vi "PART1.vi"() -> ()   [LabVIEW 2019]
uses:
  <vilib>/rvi/eio/common/nirviEmuTemplateMethod_errors.vi
  <vilib>/eio/EIONode/EIONode.xnode
  <vilib>/eio/EIOMethodNode/EIOMethodNode.xnode
panel:
  out "SDA 11":bool
  out "SDA 10":bool
  out "SDA 9":bool
  out "SDA 8":bool
  out "SDA 7":bool
  out "SDA 6":bool
  out "SDA 5":bool
  out "SDA 4":bool
  out "SDA 3":bool
  out "SDA 2":bool
  out "SDA":bool
diagram:
  n1 = flat-sequence {
    frame #0 {
      n2 = xnode "FPGA I/O Node"("SDA"=FALSE) -> ()  [unwired: 1 in, 1 out]
      n3 = xnode "FPGA I/O Node"("SCL"=TRUE) -> ()  [unwired: 1 in, 1 out]
    }
    frame #1 {
      n4 = call "Wait3"("Count(mSec)"=u32 100) -> ()  [unwired: 1 out]
    }
    frame #2 {
      n5 = xnode "FPGA I/O Node"("SCL"=FALSE) -> ()  [unwired: 1 in, 1 out]
    }
    frame #3 {
      n6 = call "Wait"("Count(mSec)"=u32 100) -> ()  [unwired: 1 out]
    }
    frame #4 {
      # "bit 0"
      n7 = xnode "FPGA I/O Node"("SDA"=FALSE) -> ()  [unwired: 1 in, 1 out]
    }
    frame #5 {
      n8 = xnode "FPGA I/O Node"("SCL"=TRUE) -> ()  [unwired: 1 in, 1 out]
    }
    frame #6 {
      n9 = call "Wait2"("Count(mSec)"=u32 100) -> ()  [unwired: 1 out]
    }
    frame #7 {
      n10 = xnode "FPGA I/O Node"("SCL"=FALSE) -> ()  [unwired: 1 in, 1 out]
    }
    frame #8 {
      n11 = call "Wait4"("Count(mSec)"=u32 100) -> ()  [unwired: 1 out]
    }
    frame #9 {
      # "bit 0"
      n12 = xnode "FPGA I/O Node"("SDA"=FALSE) -> ()  [unwired: 1 in, 1 out]
    }
    frame #10 {
      n13 = xnode "FPGA I/O Node"("SCL"=TRUE) -> ()  [unwired: 1 in, 1 out]
    }
    frame #11 {
      n14 = call "Wait6"("Count(mSec)"=u32 100) -> ()  [unwired: 1 out]
    }
    frame #12 {
      n15 = xnode "FPGA I/O Node"("SCL"=FALSE) -> ()  [unwired: 1 in, 1 out]
    }
    frame #13 {
      n16 = call "Wait5"("Count(mSec)"=u32 100) -> ()  [unwired: 1 out]
    }
    frame #14 {
      # "bit 1"
      n17 = xnode "FPGA I/O Node"("SDA"=TRUE) -> ()  [unwired: 1 in, 1 out]
    }
    frame #15 {
      n18 = xnode "FPGA I/O Node"("SCL"=TRUE) -> ()  [unwired: 1 in, 1 out]
    }
    frame #16 {
      n19 = call "Wait7"("Count(mSec)"=u32 100) -> ()  [unwired: 1 out]
    }
    frame #17 {
      n20 = xnode "FPGA I/O Node"("SCL"=FALSE) -> ()  [unwired: 1 in, 1 out]
    }
    frame #18 {
      n21 = call "Wait8"("Count(mSec)"=u32 100) -> ()  [unwired: 1 out]
    }
    frame #19 {
      # "bit 1"
      n22 = xnode "FPGA I/O Node"("SDA"=TRUE) -> ()  [unwired: 1 in, 1 out]
    }
    frame #20 {
      n23 = xnode "FPGA I/O Node"("SCL"=TRUE) -> ()  [unwired: 1 in, 1 out]
    }
    frame #21 {
      n24 = call "Wait9"("Count(mSec)"=u32 100) -> ()  [unwired: 1 out]
    }
    frame #22 {
      n25 = xnode "FPGA I/O Node"("SCL"=FALSE) -> ()  [unwired: 1 in, 1 out]
    }
    frame #23 {
      n26 = call "Wait10"("Count(mSec)"=u32 100) -> ()  [unwired: 1 out]
    }
    frame #24 {
      # "bit 0"
      n27 = xnode "FPGA I/O Node"("SDA"=FALSE) -> ()  [unwired: 1 in, 1 out]
    }
    frame #25 {
      n28 = xnode "FPGA I/O Node"("SCL"=TRUE) -> ()  [unwired: 1 in, 1 out]
    }
    frame #26 {
      n29 = call "Wait11"("Count(mSec)"=u32 100) -> ()  [unwired: 1 out]
    }
    frame #27 {
      n30 = xnode "FPGA I/O Node"("SCL"=FALSE) -> ()  [unwired: 1 in, 1 out]
    }
    frame #28 {
      n31 = call "Wait12"("Count(mSec)"=u32 100) -> ()  [unwired: 1 out]
    }
    frame #29 {
      # "bit 0"
      n32 = xnode "FPGA I/O Node"("SDA"=FALSE) -> ()  [unwired: 1 in, 1 out]
    }
    frame #30 {
      n33 = xnode "FPGA I/O Node"("SCL"=TRUE) -> ()  [unwired: 1 in, 1 out]
    }
    frame #31 {
      n34 = call "Wait13"("Count(mSec)"=u32 100) -> ()  [unwired: 1 out]
    }
    frame #32 {
      n35 = xnode "FPGA I/O Node"("SCL"=FALSE) -> ()  [unwired: 1 in, 1 out]
    }
    frame #33 {
      n36 = call "Wait14"("Count(mSec)"=u32 100) -> ()  [unwired: 1 out]
    }
    frame #34 {
      # "bit 1"
      n37 = xnode "FPGA I/O Node"("SDA"=TRUE) -> ()  [unwired: 1 in, 1 out]
    }
    frame #35 {
      n38 = xnode "FPGA I/O Node"("SCL"=TRUE) -> ()  [unwired: 1 in, 1 out]
    }
    frame #36 {
      n39 = call "Wait15"("Count(mSec)"=u32 100) -> ()  [unwired: 1 out]
    }
    frame #37 {
      n40 = xnode "FPGA I/O Node"("SCL"=FALSE) -> ()  [unwired: 1 in, 1 out]
    }
    frame #38 {
      n41 = call "Wait16"("Count(mSec)"=u32 100) -> ()  [unwired: 1 out]
    }
    frame #39 {
      # "bit 0"
      n42 = xnode "FPGA I/O Node"("SDA"=FALSE) -> ()  [unwired: 1 in, 1 out]
    }
    frame #40 {
      n43 = xnode "FPGA I/O Node"("SCL"=TRUE) -> ()  [unwired: 1 in, 1 out]
    }
    frame #41 {
      n44 = call "Wait17"("Count(mSec)"=u32 100) -> ()  [unwired: 1 out]
    }
    frame #42 {
      n45 = xnode "FPGA I/O Node"("SCL"=FALSE) -> ()  [unwired: 1 in, 1 out]
    }
    frame #43 {
      n46 = call "Wait18"("Count(mSec)"=u32 100) -> ()  [unwired: 1 out]
    }
    frame #44 {
      n47 = flat-sequence {
        frame #0 {
          n48 = xnode "FPGA I/O Method Node"("Enable"=FALSE) -> ()  [unwired: 1 in, 1 out]
        }
        frame #1 {
          # "Read ACK"
          n49 = xnode "FPGA I/O Node"() -> ("SDA"=→"SDA":bool)  [unwired: 1 in, 1 out]
        }
      }
    }
    frame #45 {
      n50 = xnode "FPGA I/O Node"("SCL"=TRUE) -> ()  [unwired: 1 in, 1 out]
    }
    frame #46 {
      n51 = call "Wait19"("Count(mSec)"=u32 100) -> ()  [unwired: 1 out]
    }
    frame #47 {
      n52 = xnode "FPGA I/O Node"("SCL"=FALSE) -> ()  [unwired: 1 in, 1 out]
    }
    frame #48 {
      n53 = call "Wait20"("Count(mSec)"=u32 100) -> ()  [unwired: 1 out]
    }
    frame #49 {
      # "bit 0"
      n54 = xnode "FPGA I/O Node"("SDA"=FALSE) -> ()  [unwired: 1 in, 1 out]
    }
    frame #50 {
      n55 = xnode "FPGA I/O Node"("SCL"=TRUE) -> ()  [unwired: 1 in, 1 out]
    }
    frame #51 {
      n56 = call "Wait21"("Count(mSec)"=u32 100) -> ()  [unwired: 1 out]
    }
    frame #52 {
      n57 = xnode "FPGA I/O Node"("SCL"=FALSE) -> ()  [unwired: 1 in, 1 out]
    }
    frame #53 {
      n58 = call "Wait22"("Count(mSec)"=u32 100) -> ()  [unwired: 1 out]
    }
    frame #54 {
      # "bit 1"
      n59 = xnode "FPGA I/O Node"("SDA"=TRUE) -> ()  [unwired: 1 in, 1 out]
    }
    frame #55 {
      n60 = xnode "FPGA I/O Node"("SCL"=TRUE) -> ()  [unwired: 1 in, 1 out]
    }
    frame #56 {
      n61 = call "Wait23"("Count(mSec)"=u32 100) -> ()  [unwired: 1 out]
    }
    frame #57 {
      n62 = xnode "FPGA I/O Node"("SCL"=FALSE) -> ()  [unwired: 1 in, 1 out]
    }
    frame #58 {
      n63 = call "Wait24"("Count(mSec)"=u32 100) -> ()  [unwired: 1 out]
    }
    frame #59 {
      # "bit 0"
      n64 = xnode "FPGA I/O Node"("SDA"=FALSE) -> ()  [unwired: 1 in, 1 out]
    }
    frame #60 {
      n65 = xnode "FPGA I/O Node"("SCL"=TRUE) -> ()  [unwired: 1 in, 1 out]
    }
    frame #61 {
      n66 = call "Wait25"("Count(mSec)"=u32 100) -> ()  [unwired: 1 out]
    }
    frame #62 {
      n67 = xnode "FPGA I/O Node"("SCL"=FALSE) -> ()  [unwired: 1 in, 1 out]
    }
    frame #63 {
      n68 = call "Wait26"("Count(mSec)"=u32 100) -> ()  [unwired: 1 out]
    }
    frame #64 {
      # "bit 1"
      n69 = xnode "FPGA I/O Node"("SDA"=TRUE) -> ()  [unwired: 1 in, 1 out]
    }
    frame #65 {
      n70 = xnode "FPGA I/O Node"("SCL"=TRUE) -> ()  [unwired: 1 in, 1 out]
    }
    frame #66 {
      n71 = call "Wait27"("Count(mSec)"=u32 100) -> ()  [unwired: 1 out]
    }
    frame #67 {
      n72 = xnode "FPGA I/O Node"("SCL"=FALSE) -> ()  [unwired: 1 in, 1 out]
    }
    frame #68 {
      n73 = call "Wait28"("Count(mSec)"=u32 100) -> ()  [unwired: 1 out]
    }
    frame #69 {
      # "bit 0"
      n74 = xnode "FPGA I/O Node"("SDA"=FALSE) -> ()  [unwired: 1 in, 1 out]
    }
    frame #70 {
      n75 = xnode "FPGA I/O Node"("SCL"=TRUE) -> ()  [unwired: 1 in, 1 out]
    }
    frame #71 {
      n76 = call "Wait29"("Count(mSec)"=u32 100) -> ()  [unwired: 1 out]
    }
    frame #72 {
      n77 = xnode "FPGA I/O Node"("SCL"=FALSE) -> ()  [unwired: 1 in, 1 out]
    }
    frame #73 {
      n78 = call "Wait30"("Count(mSec)"=u32 100) -> ()  [unwired: 1 out]
    }
    frame #74 {
      # "bit 0"
      n79 = xnode "FPGA I/O Node"("SDA"=FALSE) -> ()  [unwired: 1 in, 1 out]
    }
    frame #75 {
      n80 = xnode "FPGA I/O Node"("SCL"=TRUE) -> ()  [unwired: 1 in, 1 out]
    }
    frame #76 {
      n81 = call "Wait31"("Count(mSec)"=u32 100) -> ()  [unwired: 1 out]
    }
    frame #77 {
      n82 = xnode "FPGA I/O Node"("SCL"=FALSE) -> ()  [unwired: 1 in, 1 out]
    }
    frame #78 {
      n83 = call "Wait32"("Count(mSec)"=u32 100) -> ()  [unwired: 1 out]
    }
    frame #79 {
      # "bit 1"
      n84 = xnode "FPGA I/O Node"("SDA"=TRUE) -> ()  [unwired: 1 in, 1 out]
    }
    frame #80 {
      n85 = xnode "FPGA I/O Node"("SCL"=TRUE) -> ()  [unwired: 1 in, 1 out]
    }
    frame #81 {
      n86 = call "Wait33"("Count(mSec)"=u32 100) -> ()  [unwired: 1 out]
    }
    frame #82 {
      n87 = xnode "FPGA I/O Node"("SCL"=FALSE) -> ()  [unwired: 1 in, 1 out]
    }
    frame #83 {
      n88 = call "Wait34"("Count(mSec)"=u32 100) -> ()  [unwired: 1 out]
    }
    frame #84 {
      n89 = flat-sequence {
        frame #0 {
          n90 = xnode "FPGA I/O Method Node"("Enable"=FALSE) -> ()  [unwired: 1 in, 1 out]
        }
        frame #1 {
          # "Read ACK"
          n91 = xnode "FPGA I/O Node"() -> ("SDA"=→"SDA 2":bool)  [unwired: 1 in, 1 out]
        }
      }
    }
    frame #85 {
      n92 = xnode "FPGA I/O Node"("SDA"=FALSE) -> ()  [unwired: 1 in, 1 out]
      n93 = xnode "FPGA I/O Node"("SCL"=TRUE) -> ()  [unwired: 1 in, 1 out]
    }
    frame #86 {
      n94 = call "Wait35"("Count(mSec)"=u32 100) -> ()  [unwired: 1 out]
    }
    frame #87 {
      n95 = xnode "FPGA I/O Node"("SCL"=FALSE) -> ()  [unwired: 1 in, 1 out]
    }
    frame #88 {
      n96 = call "Wait36"("Count(mSec)"=u32 100) -> ()  [unwired: 1 out]
    }
    frame #89 {
      # "bit 0"
      n97 = xnode "FPGA I/O Node"("SDA"=FALSE) -> ()  [unwired: 1 in, 1 out]
    }
    frame #90 {
      n98 = xnode "FPGA I/O Node"("SCL"=TRUE) -> ()  [unwired: 1 in, 1 out]
    }
    frame #91 {
      n99 = call "Wait37"("Count(mSec)"=u32 100) -> ()  [unwired: 1 out]
    }
    frame #92 {
      n100 = xnode "FPGA I/O Node"("SCL"=FALSE) -> ()  [unwired: 1 in, 1 out]
    }
    frame #93 {
      n101 = call "Wait38"("Count(mSec)"=u32 100) -> ()  [unwired: 1 out]
    }
    frame #94 {
      # "bit 0"
      n102 = xnode "FPGA I/O Node"("SDA"=FALSE) -> ()  [unwired: 1 in, 1 out]
    }
    frame #95 {
      n103 = xnode "FPGA I/O Node"("SCL"=TRUE) -> ()  [unwired: 1 in, 1 out]
    }
    frame #96 {
      n104 = call "Wait39"("Count(mSec)"=u32 100) -> ()  [unwired: 1 out]
    }
    frame #97 {
      n105 = xnode "FPGA I/O Node"("SCL"=FALSE) -> ()  [unwired: 1 in, 1 out]
    }
    frame #98 {
      n106 = call "Wait40"("Count(mSec)"=u32 100) -> ()  [unwired: 1 out]
    }
    frame #99 {
      # "bit 1"
      n107 = xnode "FPGA I/O Node"("SDA"=TRUE) -> ()  [unwired: 1 in, 1 out]
    }
    frame #100 {
      n108 = xnode "FPGA I/O Node"("SCL"=TRUE) -> ()  [unwired: 1 in, 1 out]
    }
    frame #101 {
      n109 = call "Wait41"("Count(mSec)"=u32 100) -> ()  [unwired: 1 out]
    }
    frame #102 {
      n110 = xnode "FPGA I/O Node"("SCL"=FALSE) -> ()  [unwired: 1 in, 1 out]
    }
    frame #103 {
      n111 = call "Wait42"("Count(mSec)"=u32 100) -> ()  [unwired: 1 out]
    }
    frame #104 {
      # "bit 1"
      n112 = xnode "FPGA I/O Node"("SDA"=TRUE) -> ()  [unwired: 1 in, 1 out]
    }
    frame #105 {
      n113 = xnode "FPGA I/O Node"("SCL"=TRUE) -> ()  [unwired: 1 in, 1 out]
    }
    frame #106 {
      n114 = call "Wait43"("Count(mSec)"=u32 100) -> ()  [unwired: 1 out]
    }
    frame #107 {
      n115 = xnode "FPGA I/O Node"("SCL"=FALSE) -> ()  [unwired: 1 in, 1 out]
    }
    frame #108 {
      n116 = call "Wait44"("Count(mSec)"=u32 100) -> ()  [unwired: 1 out]
    }
    frame #109 {
      # "bit 0"
      n117 = xnode "FPGA I/O Node"("SDA"=FALSE) -> ()  [unwired: 1 in, 1 out]
    }
    frame #110 {
      n118 = xnode "FPGA I/O Node"("SCL"=TRUE) -> ()  [unwired: 1 in, 1 out]
    }
    frame #111 {
      n119 = call "Wait45"("Count(mSec)"=u32 100) -> ()  [unwired: 1 out]
    }
    frame #112 {
      n120 = xnode "FPGA I/O Node"("SCL"=FALSE) -> ()  [unwired: 1 in, 1 out]
    }
    frame #113 {
      n121 = call "Wait46"("Count(mSec)"=u32 100) -> ()  [unwired: 1 out]
    }
    frame #114 {
      # "bit 0"
      n122 = xnode "FPGA I/O Node"("SDA"=FALSE) -> ()  [unwired: 1 in, 1 out]
    }
    frame #115 {
      n123 = xnode "FPGA I/O Node"("SCL"=TRUE) -> ()  [unwired: 1 in, 1 out]
    }
    frame #116 {
      n124 = call "Wait47"("Count(mSec)"=u32 100) -> ()  [unwired: 1 out]
    }
    frame #117 {
      n125 = xnode "FPGA I/O Node"("SCL"=FALSE) -> ()  [unwired: 1 in, 1 out]
    }
    frame #118 {
      n126 = call "Wait48"("Count(mSec)"=u32 100) -> ()  [unwired: 1 out]
    }
    frame #119 {
      # "bit 1"
      n127 = xnode "FPGA I/O Node"("SDA"=TRUE) -> ()  [unwired: 1 in, 1 out]
    }
    frame #120 {
      n128 = xnode "FPGA I/O Node"("SCL"=TRUE) -> ()  [unwired: 1 in, 1 out]
    }
    frame #121 {
      n129 = call "Wait49"("Count(mSec)"=u32 100) -> ()  [unwired: 1 out]
    }
    frame #122 {
      n130 = xnode "FPGA I/O Node"("SCL"=FALSE) -> ()  [unwired: 1 in, 1 out]
    }
    frame #123 {
      n131 = call "Wait50"("Count(mSec)"=u32 100) -> ()  [unwired: 1 out]
    }
    frame #124 {
      # "bit 1"
      n132 = xnode "FPGA I/O Node"("SDA"=TRUE) -> ()  [unwired: 1 in, 1 out]
    }
    frame #125 {
      n133 = xnode "FPGA I/O Node"("SCL"=TRUE) -> ()  [unwired: 1 in, 1 out]
    }
    frame #126 {
      n134 = call "Wait51"("Count(mSec)"=u32 100) -> ()  [unwired: 1 out]
    }
    frame #127 {
      n135 = xnode "FPGA I/O Node"("SCL"=FALSE) -> ()  [unwired: 1 in, 1 out]
    }
    frame #128 {
      # "read ACK"
      n136 = flat-sequence {
        frame #0 {
          n137 = xnode "FPGA I/O Method Node"("Enable"=FALSE) -> ()  [unwired: 1 in, 1 out]
        }
        frame #1 {
          # "Read ACK"
          n138 = xnode "FPGA I/O Node"() -> ("SDA"=→"SDA 3":bool)  [unwired: 1 in, 1 out]
        }
      }
    }
    frame #129 {
      n139 = xnode "FPGA I/O Node"("SCL"=TRUE) -> ()  [unwired: 1 in, 1 out]
    }
    frame #130 {
      n140 = call "Wait52"("Count(mSec)"=u32 100) -> ()  [unwired: 1 out]
    }
    frame #131 {
      n141 = xnode "FPGA I/O Node"("SCL"=FALSE) -> ()  [unwired: 1 in, 1 out]
    }
    frame #132 {
      # "read MSB Data"
      n142 = xnode "FPGA I/O Node"() -> ("SDA"=→"SDA 4":bool)  [unwired: 1 in, 1 out]
    }
    frame #133 {
      n143 = xnode "FPGA I/O Node"("SCL"=TRUE) -> ()  [unwired: 1 in, 1 out]
    }
    frame #134 {
      n144 = call "Wait53"("Count(mSec)"=u32 100) -> ()  [unwired: 1 out]
    }
    frame #135 {
      n145 = xnode "FPGA I/O Node"("SCL"=FALSE) -> ()  [unwired: 1 in, 1 out]
    }
    frame #136 {
      n146 = call "Wait54"("Count(mSec)"=u32 100) -> ()  [unwired: 1 out]
    }
    frame #137 {
      # "read Data"
      n147 = xnode "FPGA I/O Node"() -> ("SDA"=→"SDA 5":bool)  [unwired: 1 in, 1 out]
    }
    frame #138 {
      n148 = xnode "FPGA I/O Node"("SCL"=TRUE) -> ()  [unwired: 1 in, 1 out]
    }
    frame #139 {
      n149 = call "Wait55"("Count(mSec)"=u32 100) -> ()  [unwired: 1 out]
    }
    frame #140 {
      n150 = xnode "FPGA I/O Node"("SCL"=FALSE) -> ()  [unwired: 1 in, 1 out]
    }
    frame #141 {
      n151 = call "Wait56"("Count(mSec)"=u32 100) -> ()  [unwired: 1 out]
    }
    frame #142 {
      # "read Data"
      n152 = xnode "FPGA I/O Node"() -> ("SDA"=→"SDA 7":bool)  [unwired: 1 in, 1 out]
    }
    frame #143 {
      n153 = xnode "FPGA I/O Node"("SCL"=TRUE) -> ()  [unwired: 1 in, 1 out]
    }
    frame #144 {
      n154 = call "Wait57"("Count(mSec)"=u32 100) -> ()  [unwired: 1 out]
    }
    frame #145 {
      n155 = xnode "FPGA I/O Node"("SCL"=FALSE) -> ()  [unwired: 1 in, 1 out]
    }
    frame #146 {
      n156 = call "Wait58"("Count(mSec)"=u32 100) -> ()  [unwired: 1 out]
    }
    frame #147 {
      # "read Data"
      n157 = xnode "FPGA I/O Node"() -> ("SDA"=→"SDA 6":bool)  [unwired: 1 in, 1 out]
    }
    frame #148 {
      n158 = xnode "FPGA I/O Node"("SCL"=TRUE) -> ()  [unwired: 1 in, 1 out]
    }
    frame #149 {
      n159 = call "Wait59"("Count(mSec)"=u32 100) -> ()  [unwired: 1 out]
    }
    frame #150 {
      n160 = xnode "FPGA I/O Node"("SCL"=FALSE) -> ()  [unwired: 1 in, 1 out]
    }
    frame #151 {
      n161 = call "Wait60"("Count(mSec)"=u32 100) -> ()  [unwired: 1 out]
    }
    frame #152 {
      # "read Data"
      n162 = xnode "FPGA I/O Node"() -> ("SDA"=→"SDA 8":bool)  [unwired: 1 in, 1 out]
    }
    frame #153 {
      n163 = xnode "FPGA I/O Node"("SCL"=TRUE) -> ()  [unwired: 1 in, 1 out]
    }
    frame #154 {
      n164 = call "Wait61"("Count(mSec)"=u32 100) -> ()  [unwired: 1 out]
    }
    frame #155 {
      n165 = xnode "FPGA I/O Node"("SCL"=FALSE) -> ()  [unwired: 1 in, 1 out]
    }
    frame #156 {
      n166 = call "Wait62"("Count(mSec)"=u32 100) -> ()  [unwired: 1 out]
    }
    frame #157 {
      # "read Data"
      n167 = xnode "FPGA I/O Node"() -> ("SDA"=→"SDA 9":bool)  [unwired: 1 in, 1 out]
    }
    frame #158 {
      n168 = xnode "FPGA I/O Node"("SCL"=TRUE) -> ()  [unwired: 1 in, 1 out]
    }
    frame #159 {
      n169 = call "Wait63"("Count(mSec)"=u32 100) -> ()  [unwired: 1 out]
    }
    frame #160 {
      n170 = xnode "FPGA I/O Node"("SCL"=FALSE) -> ()  [unwired: 1 in, 1 out]
    }
    frame #161 {
      n171 = call "Wait64"("Count(mSec)"=u32 100) -> ()  [unwired: 1 out]
    }
    frame #162 {
      # "read Data"
      n172 = xnode "FPGA I/O Node"() -> ("SDA"=→"SDA 10":bool)  [unwired: 1 in, 1 out]
    }
    frame #163 {
      n173 = xnode "FPGA I/O Node"("SCL"=TRUE) -> ()  [unwired: 1 in, 1 out]
    }
    frame #164 {
      n174 = call "Wait65"("Count(mSec)"=u32 100) -> ()  [unwired: 1 out]
    }
    frame #165 {
      n175 = xnode "FPGA I/O Node"("SCL"=FALSE) -> ()  [unwired: 1 in, 1 out]
    }
    frame #166 {
      n176 = call "Wait66"("Count(mSec)"=u32 100) -> ()  [unwired: 1 out]
    }
    frame #167 {
      # "read Data"
      n177 = xnode "FPGA I/O Node"() -> ("SDA"=→"SDA 11":bool)  [unwired: 1 in, 1 out]
    }
    frame #168 {
      n178 = xnode "FPGA I/O Node"("SCL"=TRUE) -> ()  [unwired: 1 in, 1 out]
    }
    frame #169 {
      n179 = call "Wait67"("Count(mSec)"=u32 100) -> ()  [unwired: 1 out]
    }
    frame #170 {
      n180 = xnode "FPGA I/O Node"("SCL"=FALSE) -> ()  [unwired: 1 in, 1 out]
    }
    frame #171 {
      n181 = call "Wait68"("Count(mSec)"=u32 100) -> ()  [unwired: 1 out]
    }
    frame #172 {
      # "bit 1"
      n182 = xnode "FPGA I/O Node"("SDA"=TRUE) -> ()  [unwired: 1 in, 1 out]
    }
    frame #173 {
      n183 = xnode "FPGA I/O Node"("SCL"=TRUE) -> ()  [unwired: 1 in, 1 out]
    }
    frame #174 {
      n184 = call "Wait69"("Count(mSec)"=u32 100) -> ()  [unwired: 1 out]
    }
    frame #175 {
      n185 = xnode "FPGA I/O Node"("SCL"=FALSE) -> ()  [unwired: 1 in, 1 out]
    }
    frame #176 {
      n186 = call "Wait70"("Count(mSec)"=u32 100) -> ()  [unwired: 1 out]
    }
    frame #177 {
      # "bit 0"
      n187 = xnode "FPGA I/O Node"("SDA"=FALSE) -> ()  [unwired: 1 in, 1 out]
    }
    frame #178 {
      n188 = xnode "FPGA I/O Node"("SCL"=TRUE) -> ()  [unwired: 1 in, 1 out]
    }
    frame #179 {
      n189 = call "Wait71"("Count(mSec)"=u32 100) -> ()  [unwired: 1 out]
    }
  }
